vi "Linear Algebra Calculator.vi"() -> ()   [LabVIEW 2023]
doc: "Performs a variety of linear algebra operations, such as determinant, norm, and product, on the matrix A, or in some cases, on the system of equations defined by Ax = b.\n\nNote: You must have the LabVIEW Full or Professional Development Systems to run this example."
uses:
  <vilib>/Analysis/_algsub.llb/Matrix Norm Type.ctl
  <vilib>/Analysis/7linalg.llb/Eigenvalue and Vectors Output Option.ctl
  <vilib>/Analysis/_algsub.llb/Matrix Type for Test.ctl
  <vilib>/Analysis/7linalg.llb/Real Cholesky Factorization.vi
  <vilib>/Analysis/_algsub.llb/Real Matrix Condition Number.vi
  <vilib>/Analysis/baseanly.llb/Real Determinant.vi
  <vilib>/Analysis/_algsub.llb/Real Matrix Norm.vi
  <vilib>/Analysis/_algsub.llb/Real PseudoInverse Matrix.vi
  <vilib>/Analysis/7linalg.llb/Real QR Decomposition.vi
  <vilib>/Analysis/_algsub.llb/Real Matrix Rank.vi
  <vilib>/Analysis/7linalg.llb/Solve Linear Equations (single right hand).vi
  <vilib>/Analysis/_algsub.llb/Real Matrix Trace.vi
  <vilib>/Analysis/baseanly.llb/Full Cholesky Factorization.vi
  <vilib>/Analysis/baseanly.llb/Full Real Matrix Cholesky Factorization.vi
  <vilib>/Analysis/baseanly.llb/Solve Linear Equations By Cholesky.vi
  <vilib>/Analysis/baseanly.llb/Real Matrix to Compact Array.vi
  <vilib>/Analysis/baseanly.llb/Real Compact Tri-Matrix Linear Eqs.vi
  <vilib>/Analysis/7linalg.llb/Real Eigenvalues and Vectors.vi
  <vilib>/Analysis/baseanly.llb/Real Inverse Matrix.vi
  <vilib>/Analysis/7linalg.llb/Real LU Factorization.vi
  <vilib>/Analysis/7linalg.llb/Solve Linear Eqs (General).vi
  <vilib>/Analysis/7linalg.llb/Solve Linear Eqs (Gen, single right hand).vi
  <vilib>/Analysis/7linalg.llb/Real SVD Decomposition.vi
  <vilib>/Analysis/_algsub.llb/Test Real Matrix Type.vi
  <vilib>/Analysis/NI_AALPro.lvlib
  <vilib>/Analysis/NI_AALBase.lvlib
panel:
  out "Error":string
  in  "Operation":i32(listbox)
  in  "Stop":bool
  out "Positive Definite?":bool
  in  "norm type":T1 items=["2-norm", "1-norm", "F-norm", "Inf-norm"]
  out "Results Complex":cdb[][](array[numeric]) format="%#_4g"
  out "Results Real":dbl[][](array[numeric])
  in  "b":dbl[](array[numeric])=[2.0, 12.0, 10.0]
  in  "A":dbl[][](array[numeric])=[[4.0, 2.0, -1.0], [1.0, 4.0, 1.0], [0.1, 1.0, 2.0]]
  # "Overview: Performs a variety of operations on a 2D numeric array with the Linear Algebra VIs.\nRequirements: LabVIEW Full Development System\nInstructions: \n1. Run the VI.\n2. Edit the input matrix A. Note that you can use the Tab key to move to another cell.\n3. Select the Linear Algebra Operation and view the result.\n4. Select other Operation values and view the results.\n5. Click Stop to stop the VI."
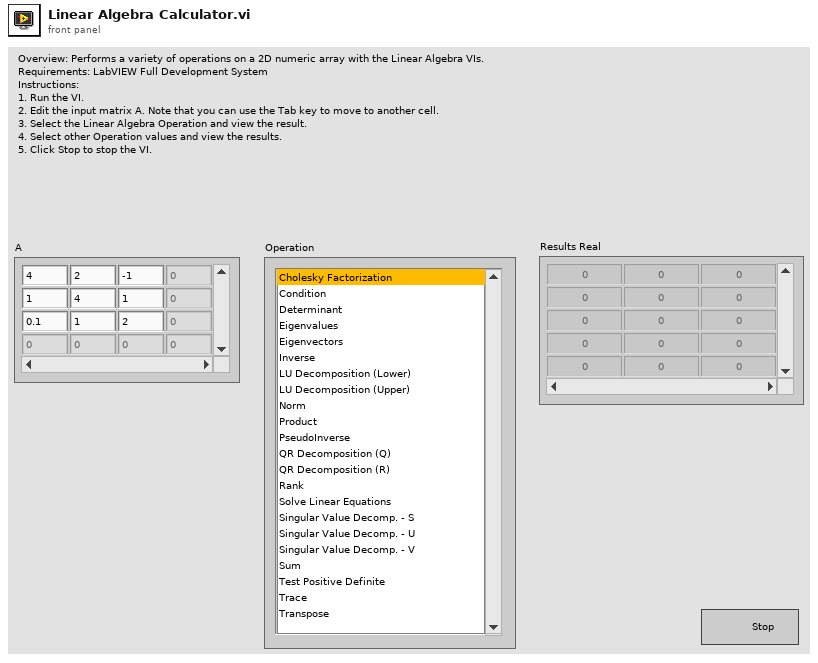
[diagram p1: front panel]
types:
  T1 = typedef "NI_AALPro.lvlib/Matrix Norm Type.ctl" = i32
  T2 = typedef "NI_Matrix.lvlib/RealMatrix.ctl" = dbl[][]
  T3 = typedef "NI_AALPro.lvlib/Eigenvalue and Vectors Output Option.ctl" = i32
  T4 = typedef "NI_Matrix.lvlib/ComplexMatrix.ctl" = cdb[][]
  T5 = typedef "NI_AALPro.lvlib/Matrix Type for Test.ctl" = i32
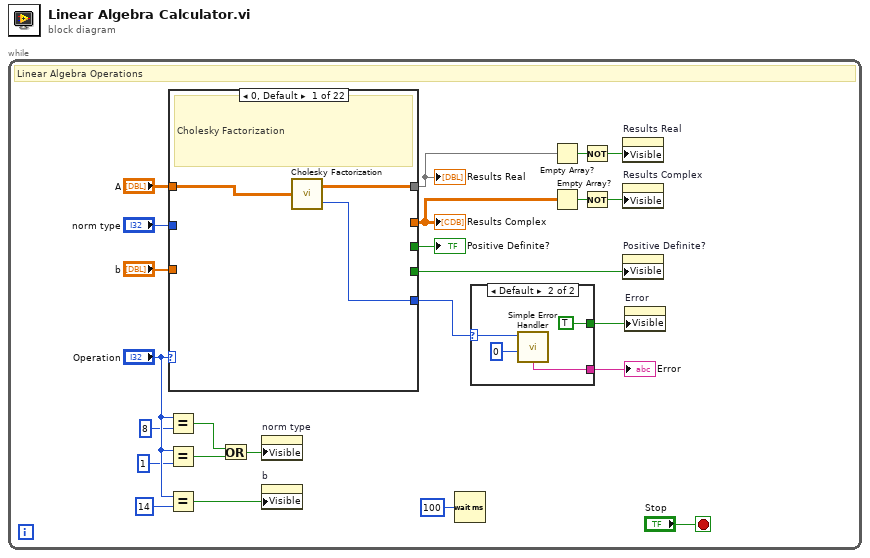
[diagram p0: block diagram]
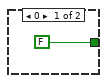
[diagram p2: hidden frame]
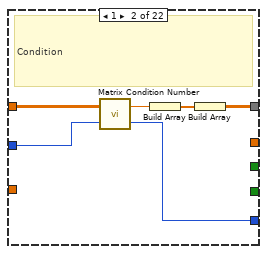
[diagram p3: hidden frame]
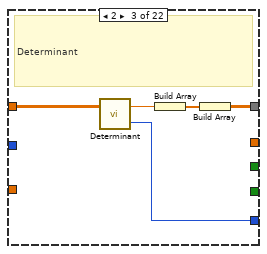
[diagram p4: hidden frame]
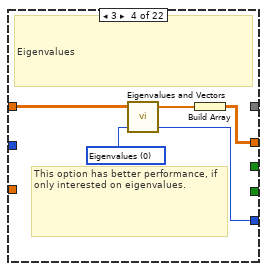
[diagram p5: hidden frame]
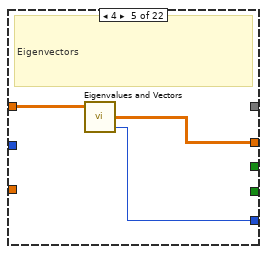
[diagram p6: hidden frame]
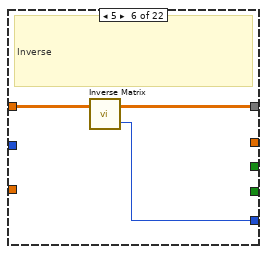
[diagram p7: hidden frame]
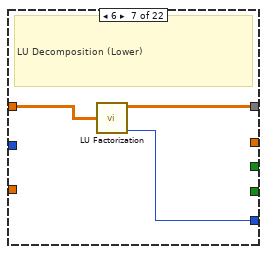
[diagram p8: hidden frame]
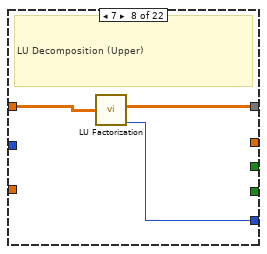
[diagram p9: hidden frame]
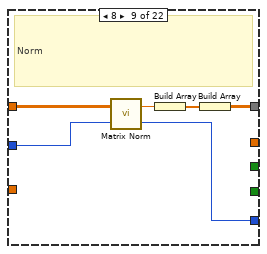
[diagram p10: hidden frame]
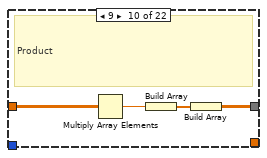
[diagram p11: hidden frame]
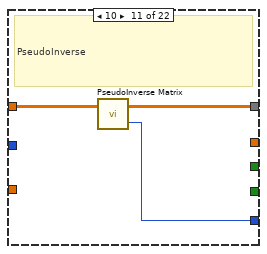
[diagram p12: hidden frame]
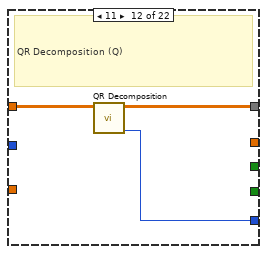
[diagram p13: hidden frame]
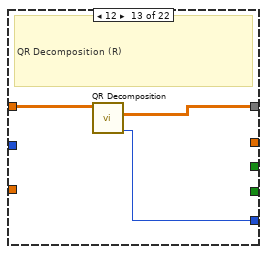
[diagram p14: hidden frame]
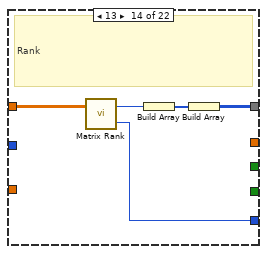
[diagram p15: hidden frame]
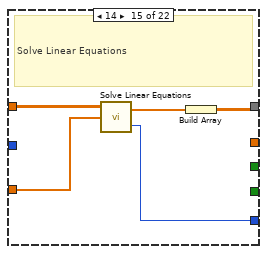
[diagram p16: hidden frame]
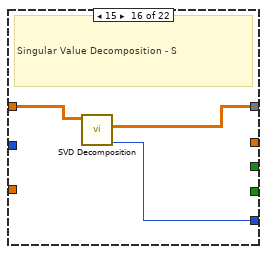
[diagram p17: hidden frame]
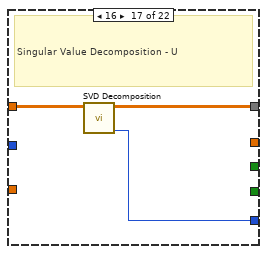
[diagram p18: hidden frame]
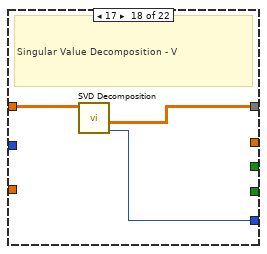
[diagram p19: hidden frame]
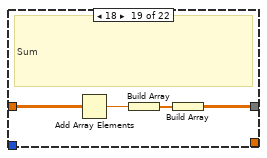
[diagram p20: hidden frame]
diagram:
  n1 = while {
    stop <- "Stop" stop-if-true
    # "Linear Algebra Operations"
    n2 = Equal?(x="Operation", y=8) -> (x = y?=w24:bool)
    n3 = Equal?(x="Operation", y=1) -> (x = y?=w19:bool)
    n4 = Equal?(x="Operation", y=14) -> (x = y?=w17:bool)
    n5 = case shown="0, Default" "Operation" {
      tunnel: "A" -> [w32 w38 w43 w48 w51 w54 w57 w60 w66 w70 w73 w76 w79 w84 w89 w92 w95 w98 w102 w107 w112 w114]
      tunnel: "b" -> [_ _ _ _ _ _ _ _ _ _ _ _ _ _ w88 _ _ _ _ _ _ _]
      tunnel: [w31 w37 w42 w47 w50 w53 w56 w59 w65 _ w72 w74 w77 w83 w87 w91 w94 w97 _ w106 w111 _] -> w2
      tunnel: "norm type" -> [_ w36 _ _ _ _ _ _ w64 _ _ _ _ _ _ _ _ _ _ _ _ _]
      tunnel: [w30 w33 w39 _ _ w52 w55 w58 w61 w67 w71 w75 w78 w80 w85 w90 w93 w96 w99 _ w108 w113] -> w16
      tunnel: [_ _ _ w45 w49 _ _ _ _ _ _ _ _ _ _ _ _ _ _ _ _ _] -> w14
      tunnel: [_ _ _ _ _ _ _ _ _ _ _ _ _ _ _ _ _ _ _ w104 _ _] -> w4
      tunnel: [_ _ _ _ _ _ _ _ _ _ _ _ _ _ _ _ _ _ _ TRUE _ _] -> w3
      frame 0, Default {
        # "Cholesky Factorization"
        n6 = call-poly <vilib>:"Cholesky Factorization.vi"("A"=w32) -> ("Cholesky"=w30:T2, "error"=w31:i32)
      }
      frame 1 {
        # "Condition"
        n7 = call-poly <vilib>:"Matrix Condition Number.vi"("norm type"=w36, "Input Matrix"=w38) -> ("error"=w37:i32, "condition number"=w35:dbl)
        n8 = Build Array(w35) -> (w34:dbl[])
        n9 = Build Array(w34) -> (w33:dbl[][])
      }
      frame 2 {
        # "Determinant"
        n10 = call-poly <vilib>:"Determinant.vi"("Input Matrix"=w43) -> ("error"=w42:i32, "determinant"=w40:dbl)  [unwired: 1 in]
        n11 = Build Array(w40) -> (w41:dbl[])
        n12 = Build Array(w41) -> (w39:dbl[][])
      }
      frame 3 {
        w44 = T3 0 items=["Eigenvalues", "Eigenvalues & Vectors"] ("output option")
        # "This option has better performance, if only interested on eigenvalues."
        # "Eigenvalues"
        n13 = call-poly <vilib>:"Eigenvalues and Vectors.vi"("output option"=w44, "Input Matrix"=w48) -> ("error"=w47:i32, "Eigenvalues"=w46:cdb[])  [unwired: 1 in, 1 out]
        n14 = Build Array(w46) -> (w45:T4)
      }
      frame 4 {
        # "Eigenvectors"
        n15 = call-poly <vilib>:"Eigenvalues and Vectors.vi"("Input Matrix"=w51) -> ("error"=w50:i32, "Eigenvectors"=w49:T4)  [unwired: 2 in, 1 out]
      }
      frame 5 {
        # "Inverse"
        n16 = call-poly <vilib>:"Inverse Matrix.vi"("Input Matrix"=w54) -> ("error"=w53:i32, "Inverse Matrix"=w52:T2)  [unwired: 1 in]
      }
      frame 6 {
        # "LU Decomposition (Lower)"
        n17 = call-poly <vilib>:"LU Factorization.vi"("A"=w57) -> ("L"=w55:T2, "error"=w56:i32)  [unwired: 2 out]
      }
      frame 7 {
        # "LU Decomposition (Upper)"
        n18 = call-poly <vilib>:"LU Factorization.vi"("A"=w60) -> ("U"=w58:T2, "error"=w59:i32)  [unwired: 2 out]
      }
      frame 8 {
        # "Norm"
        n19 = call-poly <vilib>:"Matrix Norm.vi"("norm type"=w64, "Input Matrix"=w66) -> ("error"=w65:i32, "norm"=w62:dbl)
        n20 = Build Array(w62) -> (w63:dbl[])
        n21 = Build Array(w63) -> (w61:dbl[][])
      }
      frame 9 {
        # "Product"
        n22 = Multiply Array Elements(1:w70) -> (0:w68:dbl)
        n23 = Build Array(w68) -> (w69:dbl[])
        n24 = Build Array(w69) -> (w67:dbl[][])
      }
      frame 10 {
        # "PseudoInverse"
        n25 = call-poly <vilib>:"PseudoInverse Matrix.vi"("Input Matrix"=w73) -> ("error"=w72:i32, "PseudoInverse Matrix"=w71:T2)  [unwired: 1 in]
      }
      frame 11 {
        # "QR Decomposition (Q)"
        n26 = call-poly <vilib>:"QR Decomposition.vi"("A"=w76) -> ("error"=w74:i32, "Q"=w75:T2)  [unwired: 7 in, 2 out]
      }
      frame 12 {
        # "QR Decomposition (R)"
        n27 = call-poly <vilib>:"QR Decomposition.vi"("A"=w79) -> ("error"=w77:i32, "R"=w78:T2)  [unwired: 7 in, 2 out]
      }
      frame 13 {
        # "Rank"
        n28 = call-poly <vilib>:"Matrix Rank.vi"("Input Matrix"=w84) -> ("error"=w83:i32, "rank"=w81:i32)  [unwired: 1 in]
        n29 = Build Array(w81) -> (w82:i32[])
        n30 = Build Array(w82) -> (w80:i32[][])
      }
      frame 14 {
        # "Solve Linear Equations"
        n31 = call-poly <vilib>:"Solve Linear Equations.vi"("Known Vector"=w88, "Input Matrix"=w89) -> ("error"=w87:i32, "Solution Vector"=w86:dbl[])  [unwired: 1 in]
        n32 = Build Array(w86) -> (w85:T2)
      }
      frame 15 {
        # "Singular Value Decomposition - S"
        n33 = call-poly <vilib>:"SVD Decomposition.vi"("A"=w92) -> ("error"=w91:i32, "Matrix S"=w90:T2)  [unwired: 6 in, 3 out]
      }
      frame 16 {
        # "Singular Value Decomposition - U"
        n34 = call-poly <vilib>:"SVD Decomposition.vi"("A"=w95) -> ("error"=w94:i32, "Matrix U"=w93:T2)  [unwired: 6 in, 3 out]
      }
      frame 17 {
        # "Singular Value Decomposition - V"
        n35 = call-poly <vilib>:"SVD Decomposition.vi"("A"=w98) -> ("error"=w97:i32, "Matrix V"=w96:T2)  [unwired: 6 in, 3 out]
      }
      frame 18 {
        # "Sum"
        n36 = Add Array Elements(numeric array=w102) -> (sum=w101:dbl)
        n37 = Build Array(w101) -> (w100:dbl[])
        n38 = Build Array(w100) -> (w99:dbl[][])
      }
      frame 19 {
        w105 = T5 10 items=["Symmetric Positive Definite"=10, "Symmetric Positive Semi-Definite"=11, "Symmetric"=20, "Hermitian"=21] ("matrix type")
        # "Test Positive Definite"
        n39 = call-poly <vilib>:"Test Matrix Type.vi"("matrix type"=w105, "Input Matrix"=w107) -> ("error"=w106:i32, "is type?"=w104:bool)  [unwired: 8 in]
      }
      frame 20 {
        # "Trace"
        n40 = call-poly <vilib>:"Trace.vi"("Input Matrix"=w112) -> ("trace"=w110:dbl, "error"=w111:i32)
        n41 = Build Array(w110) -> (w109:dbl[])
        n42 = Build Array(w109) -> (w108:dbl[][])
      }
      frame 21 {
        # "Transpose"
        n43 = Transpose 2D Array(2D array=w114) -> (transposed array=w113:dbl[][])
      }
    }
    "Results Real" <- w16
    "Results Complex" <- w14
    "Positive Definite?" <- w4
    n44 = Or(x=w24, y=w19) -> (x .or. y?=w20:bool)
    n45 = property on="norm type" class="Ring (strict)"("Visible"=w20) -> ()  [unwired: 2 in, 2 out]
    n46 = property on="b" class="Arr (strict)"("Visible"=w17) -> ()  [unwired: 2 in, 2 out]
    n47 = Wait (ms)(milliseconds to wait=u32 100) -> ()  [unwired: 1 out]
    n48 = case shown="Default" w2 {
      selector: w2 -> [_ w28]
      tunnel: [_ w29] -> w9
      tunnel: [FALSE TRUE] -> w8
      frame 0 {
      }
      frame Default {
        n49 = call <vilib>:"Simple Error Handler.vi"("error code (no error:0)"=w28, "type of dialog (OK msg:1)"=0) -> ("message"=w29:string)  [unwired: 3 in, 4 out]
      }
    }
    "Error" <- w9
    n50 = Empty Array?(array=w16) -> (empty?=w15:bool)
    n51 = Empty Array?(array=w14) -> (empty?=w13:bool)
    n52 = Not(x=w15) -> (.not. x?=w12:bool)
    n53 = Not(x=w13) -> (.not. x?=w11:bool)
    n54 = property on="Results Real" class="Arr (strict)"("Visible"=w12) -> ()  [unwired: 2 in, 2 out]
    n55 = property on="Results Complex" class="Arr (strict)"("Visible"=w11) -> ()  [unwired: 2 in, 2 out]
    n56 = property on="Positive Definite?" class="Bool (strict)"("Visible"=w3) -> ()  [unwired: 2 in, 2 out]
    n57 = property on="Error" class="Str"("Visible"=w8) -> ()  [unwired: 2 in, 2 out]
  }
